vi "Save Settings to XML.vi"(8 "error in (no error)":errorcluster, 11 "Settings":T1={"Support"={"Save Configuration"={"Log File Base Path"=path "", "TDMS File Reference"=refnum, "Reset"=FALSE, "Wait"=0.0, "Start Time"=0.0, "Update Rate"=0, "Channel Names"=[], "System Preset"=variant(cluster{"DB UDL file":path, "connection reference":refnum<k1>, "Writer Queue":refnum<queue>} {"DB UDL file"=path "", "connection reference"=refnum, "Writer Queue"=refnum})}, "LOG Configuration"={"LOG REF"=refnum, "Writer Queue"=refnum, "Log Path"=path "", "LOG"=FALSE}, "ALARM Configuration"={"LOG REF"=refnum, "Writer Queue"=refnum, "Log Path"=path "", "UPS standby"=FALSE, "status code"=5001, "SP"=[], "Over Sens Status"=[]}, "User Details"=[], "Radome Type"="", "Timer Configuration"={"Wait"=0.0, "Next Step"="", "Writer Queue"=refnum, "Reset"=FALSE, "VISA resource"="", "Status"=[], "Valve Time"=[], "Timer queue"=refnum, "Current valve"=0, "Enable"=FALSE}}, "Process"={"Test Configuration"={"current Step"=0, "Wait"=0.0, "Next Step"="", "Writer Queue"=refnum, "Reset"=FALSE, "SEQ Time"=0, "General Reset"=FALSE, "Cycles"=1, "Status"=[], "Ready"=[], "Backward"=FALSE, "Current SP"=[], "System Preset"={"Test Configuration"={"Cycles"=0, "Z Up"=0.0, "SP List"=[[0.0, 0.0, 0.0]], "Operator"="", "Point Delay"=0, "Z Up 2"=0.0, "Cleaning In"=0.0, "Cleaning Out"=0.0, "Cleaning Cycles"=0}, "Test_Start_date"=""}, "Test Type"=enum."Calibration", "Sample Count"=0, "Local Queues"={"Cycles queue"=refnum, "Step queue"=refnum, "RES Queue"=refnum, "Clean queue"=refnum, "PS Scan queue"=refnum}, "current Clean"=0, "PS Measure Plan"=[]}}, "Report Configuration"={"Test Setting"={"Test_Num"=5800, "Test_ID"=0, "Proc_ID"=0, "Max Force"=0.0, "User"="", "SN"="", "Date"=""}, "Measurements"=[], "LOG REF"=refnum, "Report Template"=path "", "Save Report path"=path "", "Data File Path"=path "", "Popup Dialog"=FALSE}, "History Data"={"Tests"=[], "Test Name"=""}, "Motor Configuration"={"Tango HW"={"VISA resource"="", "Baud Rate (115200)"=0, "lAnInterfaceType"=0, "bAShowProt"=0}, "Writer Queue"=refnum, "Status"=FALSE, "Abs Position"=[], "Axis Velocity"={"dX"=0.0, "dY"=0.0, "dZ"=0.0, "dA"=0.0}, "acceleration "=0.0, "Z direction"=enum."Up", "Position Mode"="", "plLSID"=0}, "PalmSense  Configuration"={"PalmSens.lvclass"=refnum, "Writer Queue"=refnum, "Enable"=FALSE, "Is Measuring Ref"=refnum, "Method"={"Name"="", "Method Ref"=variant}, "PS Live Curve Result"=refnum}, "Hiden Scanner Resources"={"Link"={"Connection"=enum."USB", "Host or IP address (TCP/IP)"="", "Port (Serial/USB)"="COM1"}, "VISA resource"="", "Writer Queue"=refnum, "Status"=FALSE}, "MFC Configuration"={"MFC Definition"={"MFC Port"="", "MFC Enable"=TRUE, "Baud Rate"=0, "Interface type"=enum."RS-485", "Address"=0}, "Set Point Options"={"Setpoint Value"=0.0, "Mass Flow EU 2"="", "Setpoint Source"="", "Valve Mode"=""}, "Writer Queue"=refnum, "Enable"=FALSE, "Update Rate"=0, "MRC Chamber Enable"=FALSE, "Selected Gas"="", "Address String"=""}} {"MFC Configuration"."Set Point Options"."Setpoint Value" min=0.0 max=0.62495 format="%.5f"; "Process"."Test Configuration"."PS Measure Plan" items=["Pretreatment settings (PS)", "Linear Sweep Voltammetry (LSV)", "Differential Pulse Voltammetry (DPV)", "Cyclic Voltammetry (CV)", "Chronoamperometry (CA)", "Chronopotentiometry (CP)", "El Imp Spectroscopy (EIS)"]; "Process"."Test Configuration"."System Preset"."Test Configuration"."SP List" format="%#.1g"; "Support"."Save Configuration"."Update Rate" min=1 max=10 step=1}) -> (0 "error out":errorcluster)   [LabVIEW 2020, in "Settings.lvlib"]
doc: "Saves the \"User Specified\" configuration data to an XML file. This is used to remember the users settings between executions."
uses:
  Settings.lvlib
  Settings.ctl
  <instrlib>/PalmSens SDK for LabVIEW 5.10/PalmSens/PalmSens.lvclass
  Logging/Save Configuration.ctl
  LOG/LOG Configuration.ctl
  support/Message Queue/Message Cluster.ctl
  ALARM/ALARM Configuration.ctl
  Valve Control/AM Configuration.ctl
  Test Driver/Test Driver Configuration.ctl
  Test Driver/System Preset.ctl
  Test Driver/Test Type.ctl
  Report/REP Configuration.ctl
  Report/Test Setting.ctl
  MOTOR/PS Hardware Configuration.ctl
  DMM/PalmSense Hardware Configuration.ctl
  Hiden Scanner/Scanner Hardware Configuration.ctl
  MRC/MRC Configuration.ctl
  <vilib>/Utility/xml.llb/Write to XML File(string).vi
  Logging/SAVE.lvlib
  LOG/LOG.lvlib
  ALARM/QCT ALARM.lvlib
  support/Message Queue/Message Queue.lvlib
  Report/Report.lvlib
  Test Driver/Test Driver.lvlib
  MOTOR/MOTOR.lvlib
  DMM/PalmSens.lvlib
  Valve Control/Valve Control.lvlib
  Hiden Scanner/Hiden Scanner.lvlib
  MRC/MRC Module.lvlib
panel:
  # "X"
  # "Y"
  # "Cycles"
  # "Point Delay"
  # "Up"
  # "Down"
  # "Z Axes"
  # "#C"
  # "In"
  # "Out"
  # "Cleaning [sec]"
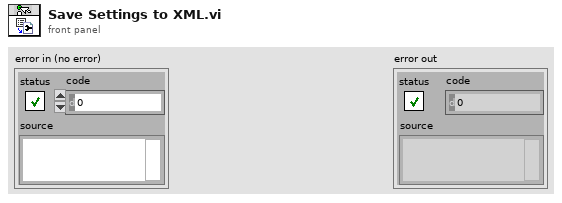
[diagram p1: front panel]
types:
  T1 = typedef "Settings.lvlib/Settings.ctl" = cluster{"Support":cluster{"Save Configuration":T2, "LOG Configuration":T3, "ALARM Configuration":T4, "User Details":string[], "Radome Type":string, "Timer Configuration":T5}, "Process":cluster{"Test Configuration":T6}, "Report Configuration":T9, "History Data":cluster{"Tests":string[][], "Test Name":string}, "Motor Configuration":T11, "PalmSense  Configuration":T12, "Hiden Scanner Resources":T13, "MFC Configuration":T14}
  T2 = typedef "SAVE.lvlib/Save Configuration.ctl" = cluster{"Log File Base Path":path, "TDMS File Reference":refnum<k34>, "Reset":bool, "Wait":dbl, "Start Time":dbl, "Update Rate":u16, "Channel Names":string[], "System Preset":variant}
  T3 = typedef "LOG.lvlib/LOG Configuration.ctl" = cluster{"LOG REF":refnum<vi>, "Writer Queue":refnum<queue>, "Log Path":path, "LOG":bool}
  T4 = typedef "QCT ALARM.lvlib/ALARM Configuration.ctl" = cluster{"LOG REF":refnum<vi>, "Writer Queue":refnum<queue>, "Log Path":path, "UPS standby":bool, "status code":i32, "SP":dbl[], "Over Sens Status":dbl[]}
  T5 = typedef "Valve Control.lvlib/AM Configuration.ctl" = cluster{"Wait":dbl, "Next Step":string, "Writer Queue":refnum<queue>, "Reset":bool, "VISA resource":refnum<visa-resource-name>, "Status":bool[], "Valve Time":dbl[], "Timer queue":refnum<queue>, "Current valve":i32, "Enable":bool}
  T6 = typedef "Test Driver.lvlib/Test Driver Configuration.ctl" = cluster{"current Step":i32, "Wait":dbl, "Next Step":string, "Writer Queue":refnum<queue>, "Reset":bool, "SEQ Time":i32, "General Reset":bool, "Cycles":i32, "Status":bool[], "Ready":bool[], "Backward":bool, "Current SP":dbl[], "System Preset":T7, "Test Type":T8, "Sample Count":i32, "Local Queues":cluster{"Cycles queue":refnum<queue>, "Step queue":refnum<queue>, "RES Queue":refnum<queue>, "Clean queue":refnum<queue>, "PS Scan queue":refnum<queue>}, "current Clean":i32, "PS Measure Plan":u16[]}
  T7 = typedef "System Preset.ctl" = cluster{"Test Configuration":cluster{"Cycles":i32, "Z Up":dbl, "SP List":dbl[][], "Operator":string, "Point Delay":i32, "Z Up 2":dbl, "Cleaning In":dbl, "Cleaning Out":dbl, "Cleaning Cycles":i32}, "Test_Start_date":string}
  T8 = typedef "Test Driver.lvlib/Test Type.ctl" = enum16{"Calibration", "Test"}
  T9 = typedef "Report.lvlib/REP Configuration.ctl" = cluster{"Test Setting":T10, "Measurements":string[][], "LOG REF":refnum<vi>, "Report Template":path, "Save Report path":path, "Data File Path":path, "Popup Dialog":bool}
  T10 = typedef "Report.lvlib/Test Setting.ctl" = cluster{"Test_Num":i32, "Test_ID":i32, "Proc_ID":i32, "Max Force":dbl, "User":string, "SN":string, "Date":string}
  T11 = typedef "MOTOR.lvlib/PS Hardware Configuration.ctl" = cluster{"Tango HW":cluster{"VISA resource":refnum<visa-resource-name>, "Baud Rate (115200)":i32, "lAnInterfaceType":i32, "bAShowProt":i32}, "Writer Queue":refnum<queue>, "Status":bool, "Abs Position":i32[], "Axis Velocity":cluster{"dX":dbl, "dY":dbl, "dZ":dbl, "dA":dbl}, "acceleration ":dbl, "Z direction":enum16{"Up", "Down"}, "Position Mode":string, "plLSID":i32}
  T12 = typedef "PalmSens.lvlib/PalmSense Hardware Configuration.ctl" = cluster{"PalmSens.lvclass":refnum<class "PalmSens.lvclass">, "Writer Queue":refnum<queue>, "Enable":bool, "Is Measuring Ref":refnum<vi>, "Method":cluster{"Name":string, "Method Ref":variant}, "PS Live Curve Result":refnum<vi>}
  T13 = typedef "Hiden Scanner.lvlib/Scanner Hardware Configuration.ctl" = cluster{"Link":cluster{"Connection":enum16{"Serial", "TCP/IP", "USB"}, "Host or IP address (TCP/IP)":string, "Port (Serial/USB)":string}, "VISA resource":refnum<visa-resource-name>, "Writer Queue":refnum<queue>, "Status":bool}
  T14 = typedef "MRC Module.lvlib/MRC Configuration.ctl" = cluster{"MFC Definition":cluster{"MFC Port":refnum<visa-resource-name>, "MFC Enable":bool, "Baud Rate":i32, "Interface type":enum32{"RS-485", "RS-232"}, "Address":i32}, "Set Point Options":cluster{"Setpoint Value":dbl, "Mass Flow EU 2":string, "Setpoint Source":string, "Valve Mode":string}, "Writer Queue":refnum<queue>, "Enable":bool, "Update Rate":u32, "MRC Chamber Enable":bool, "Selected Gas":string, "Address String":string}
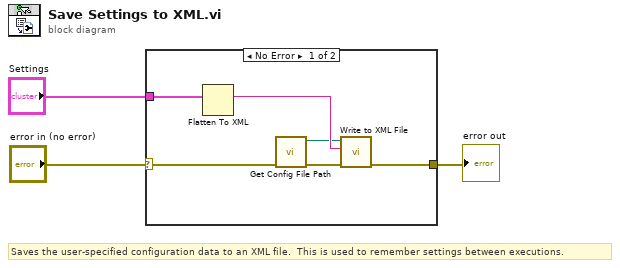
[diagram p0: block diagram]
diagram:
  # "Saves the user-specified configuration data to an XML file.  This is used to remember settings between executions."
  n1 = case shown="No Error" "error in (no error)" {
    selector: "error in (no error)" -> [w5 w10]
    tunnel: [w7 w10] -> w2
    tunnel: "Settings" -> [w9 _]
    frame No Error {
      n2 = Flatten To XML(6:w9) -> (2:w8:string)
      n3 = call "Get Config File Path.vi"("error in (no error)"=w5) -> ("error out"=w4:errorcluster, "XML File Path"=w6:path)  [unwired: 9 in]
      n4 = call-poly <vilib>:"Write to XML File.vi"("error in (no error)"=w4, "XML Input"=w8, "XML File Path"=w6) -> ("error out"=w7:errorcluster)  [unwired: 6 in, 2 out]
    }
    frame Error {
    }
  }
  "error out" <- w2
